vi "Create Reference Queue.vi"(6 "Timeout (s)":dbl, 8 "error in (no error)":errorcluster, 11 "Name":string) -> (0 "error out":errorcluster, 3 "QDMH out":refnum<class "QDMH.lvclass">)   [LabVIEW 2023, in "QDMH.lvlib" / "QDMH.lvclass"]
doc: "This utility searches for a named queue reference and returns a queue reference. \n\nThis allows external devices to access the named DQMH to hook in externally."
uses:
  Library/QDMH.lvclass
  Custom Controls/Message.ctl
  Library/QDMH.lvclass/QDMH.ctl
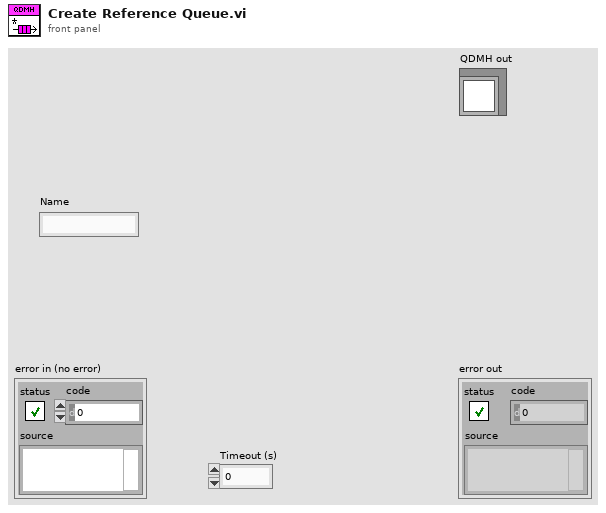
[diagram p1: front panel]
types:
  T1 = typedef "QDMH.lvlib/QDMH.lvclass/Message.ctl" = cluster{"State":string, "Data":variant}
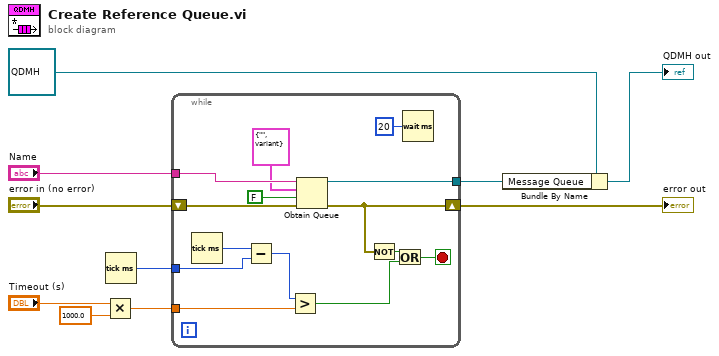
[diagram p0: block diagram]
diagram:
  n1 = Multiply(x="Timeout (s)", y=1000.0 ("x")) -> (x*y=w4:dbl)
  n2 = Tick Count (ms)() -> (millisecond timer value=w6:u32)
  n3 = while {
    tunnel: "Name" -> [w23]
    tunnel: w6 -> [w20]
    shift-right: [w12] -> w3
    shift-left: "error in (no error)" -> [w19]
    tunnel: [w18] -> w1
    tunnel: w4 -> [w15]
    stop <- w17 stop-if-true
    n4 = Tick Count (ms)() -> (millisecond timer value=w21:u32)
    n5 = Subtract(x=w21, y=w20) -> (x-y=w16:u32)
    n6 = Greater?(x=w16, y=w15) -> (0:w14:bool)
    n7 = Obtain Queue(name (unnamed)=w23, element data type=T1 {"State"="", "Data"=variant} ("Message"), create if not found? (T)=FALSE, error in (no error)=w19) -> (queue out=w18:refnum<queue>, error out=w12:errorcluster)  [unwired: 1 in, 1 out]
    n8 = Not(x=w12) -> (.not. x?=w13:bool)
    n9 = Or(x=w13, y=w14) -> (x .or. y?=w17:bool)
    n10 = Wait (ms)(milliseconds to wait=u32 20) -> ()  [unwired: 1 out]
  }
  "error out" <- w3
  n11 = Bundle By Name(cluster=refnum<class "QDMH.lvclass"> refnum ("QDMH in"), "Message Queue"=w1) -> (→"QDMH out":refnum<class "QDMH.lvclass">)
